vi "Mono (YJ) GratingJose.vi"(5 "error in (no error)":errorcluster, 7 "Go to Wavelength":dbl) -> (0 "Current Grating":string, 1 "State of Mono_SetWavelength":bool=TRUE, 2 "error out 2":errorcluster, 3 "Current Wavelength":dbl)   [LabVIEW 2017]
uses:
  C:/Users/Admin/Desktop/Sensitive EQE Stuff/S-EQE (YJ)/Mono vi (YJ)/Cornerstone.dll
  Cornerstone.dll
panel:
  in  "CmdLib In":refnum<k24>
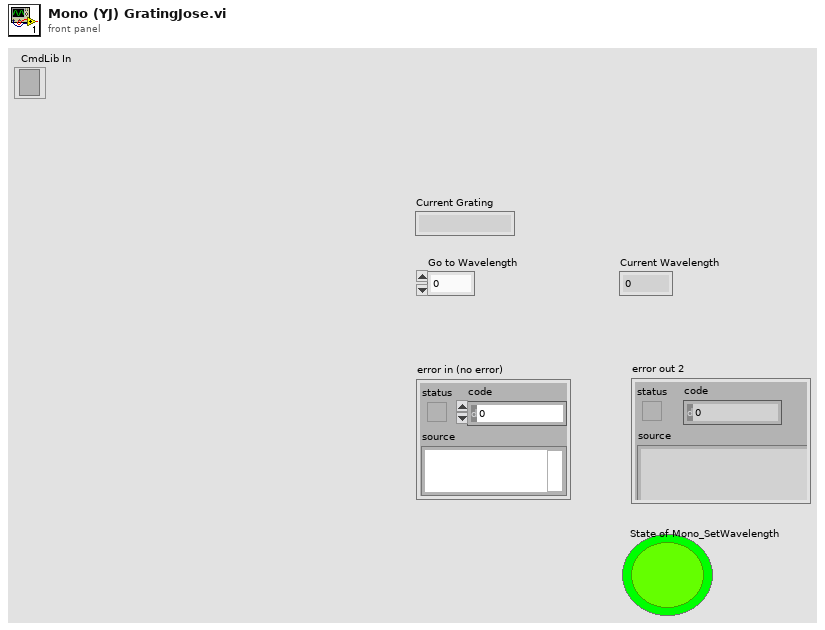
[diagram p1: front panel]
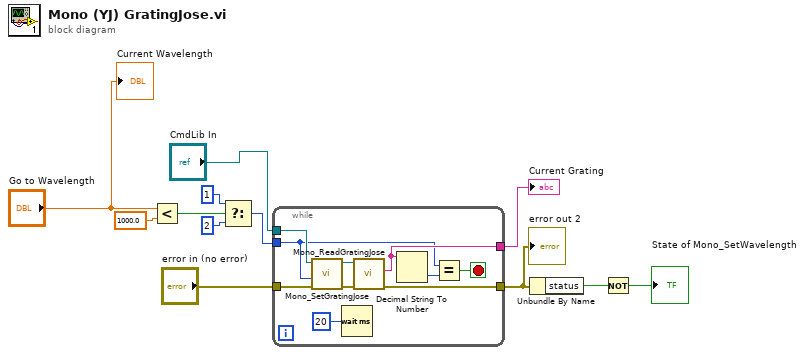
[diagram p0: block diagram]
diagram:
  n1 = Less?(x="Go to Wavelength", y=1000.0) -> (x < y?=w9:bool)
  n2 = Select(t=1 ("Grating"), s=w9, f=2) -> (s? t:f=w2:i32)
  n3 = while {
    tunnel: "CmdLib In" -> [w22]
    tunnel: [w18] -> w3
    tunnel: w2 -> [w17]
    tunnel: "error in (no error)" -> [w21]
    tunnel: [w19] -> w4
    stop <- w15 stop-if-true
    n4 = call "Mono_SetGratingJose.vi"("error in (no error) 2"=w21, "Grating"=w17, "CmdLib In"=w22) -> ("error out 2"=w20:errorcluster, "CmdLib Out"=w13:refnum<k24>)  [unwired: 6 in, 1 out]
    n5 = Wait (ms)(milliseconds to wait=u32 20) -> ()  [unwired: 1 out]
    n6 = call "Mono_ReadGratingJose.vi"("error in (no error) 2"=w20, "CmdLib In"=w13) -> ("error out 2"=w19:errorcluster, "Current Grating"=w18:string)  [unwired: 7 in, 1 out]
    n7 = Decimal String To Number(string=w18) -> (number=w16:i32)  [unwired: 2 in, 1 out]
    n8 = Equal?(x=w17, y=w16) -> (x = y?=w15:bool)
  }
  "error out 2" <- w4
  "Current Grating" <- w3
  n9 = Unbundle By Name(w4) -> ("status"=w12:bool)
  n10 = Not(x=w12) -> (.not. x?=→"State of Mono_SetWavelength":bool)
  "Current Wavelength" <- "Go to Wavelength"
